vi "NodetoID.vi"(8 "error in":errorcluster, 11 "node ref":T1) -> (0 "error out":errorcluster, 3 "ID":string)   [LabVIEW 2013, in "NISE_CEF_Node.lvclass"]
doc: "This VI cast the creates an id number for a node reference"
uses:
  NISE_CEF_Node.lvclass
  NodeRef.ctl
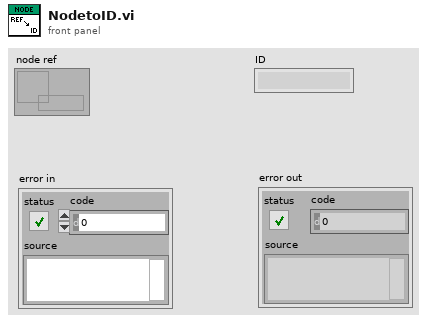
[diagram p1: front panel]
types:
  T1 = typedef "NISE_CEF_Node.lvclass/NodeRef.ctl" = refnum<data-value>
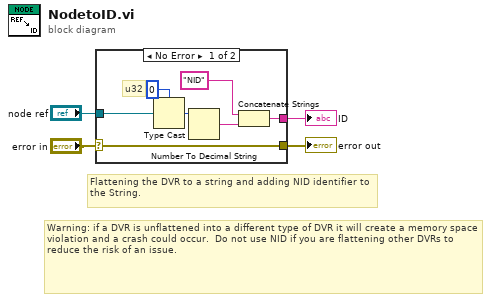
[diagram p0: block diagram]
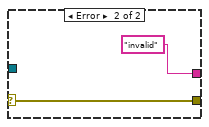
[diagram p2: hidden frame]
diagram:
  # "Warning: if a DVR is unflattened into a different type of DVR it will create a memory space violation and a crash could occur.  Do not use NID if you are flattening other DVRs to reduce the risk of an issue."
  # "Flattening the DVR to a string and adding NID identifier to the String."
  n1 = case shown="No Error" "error in" {
    selector: "error in" -> [w7 w12]
    tunnel: [w11 "invalid"] -> w4
    tunnel: "node ref" -> [w9 _]
    tunnel: [w7 w12] -> w2
    frame No Error {
      # "u32"
      n2 = Type Cast(type=u32 0, x=w9) -> (*(type *) &x=w6:u32)
      n3 = Number To Decimal String(number=w6) -> (decimal integer string=w5:string)  [unwired: 1 in]
      n4 = Concatenate Strings("NID" ("string"), w5) -> (w11:string)
    }
    frame Error {
    }
  }
  "ID" <- w4
  "error out" <- w2
